vi "Get Plot visiblity.vi"(11 "Graph_refs":T2) -> (3 "Plot visibility":T1[](array[typedef]))   [LabVIEW 2018]
uses:
  Scope/controls/Graph_references.ctl
  Scope/controls/graph_controls.ctl
  Scope/controls/Plot visibility.ctl
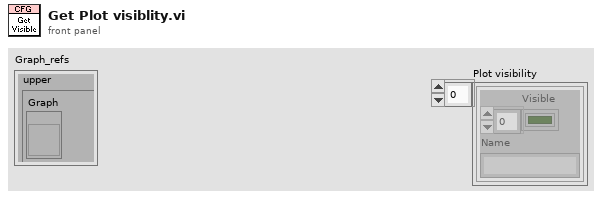
[diagram p1: front panel]
types:
  T1 = typedef "Plot visibility.ctl" = cluster{"Visible":bool[], "Name":string}
  T2 = typedef "Graph_references.ctl" = cluster{"upper":T3, "lower":T3, "Freq graph":refnum<vi>, "Adaptive FF graph":refnum<vi>}
  T3 = typedef "graph_controls.ctl" = cluster{"Graph":refnum<vi>, "Time btn":refnum<vi>, "Amplitude btn":refnum<vi>, "Chart":refnum<vi>}
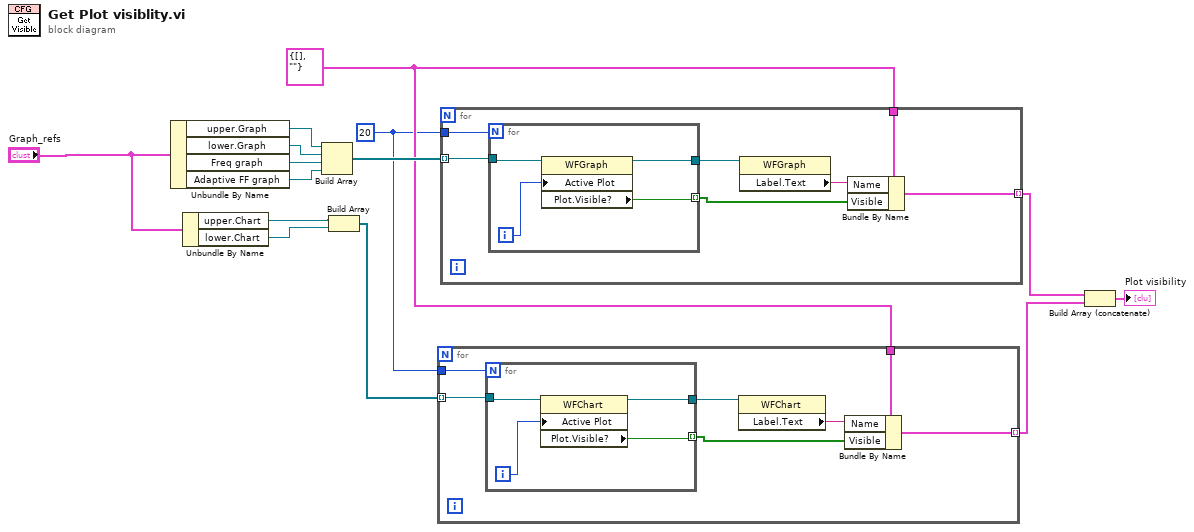
[diagram p0: block diagram]
diagram:
  w1 = 20
  w5 = T1 {"Visible"=[], "Name"=""} ("Plot visiblility")
  n1 = Unbundle By Name("Graph_refs") -> ("upper.Graph"=w14:refnum<vi>, "lower.Graph"=w13:refnum<vi>, "Freq graph"=w11:refnum<vi>, "Adaptive FF graph"=w10:refnum<vi>)
  n2 = Unbundle By Name("Graph_refs") -> ("upper.Chart"=w8:refnum<vi>, "lower.Chart"=w7:refnum<vi>)
  n3 = Build Array(w14, w13, w11, w10) -> (w12:refnum<vi>[])
  n4 = Build Array(w8, w7) -> (w6:refnum<vi>[])
  n5 = for {
    tunnel: w6 -> [w21] mode=indexing
    tunnel: w5 -> [w19]
    tunnel: [w16] -> w3 mode=indexing
    tunnel: w1 -> [w15]
    n6 = for {
      N: w15 -> [_]
      tunnel: w21 -> [w25]
      tunnel: [w23] -> w17 mode=indexing
      tunnel: [w22] -> w20
      i -> [w24]
      n7 = property on="Property Node" class="WFChart"(reference=w25, "Active Plot"=w24) -> (reference out=w22:refnum<vi>, "Plot.Visible?"=w23:bool)  [unwired: 1 in, 1 out]
    }
    n8 = property on="Property Node" class="WFChart"(reference=w20) -> ("Label.Text"=w18:string)  [unwired: 1 in, 2 out]
    n9 = Bundle By Name(cluster=w19, "Name"=w18, "Visible"=w17) -> (w16:T1)
  }
  n10 = for {
    tunnel: w12 -> [w32] mode=indexing
    tunnel: w5 -> [w30]
    tunnel: [w27] -> w4 mode=indexing
    tunnel: w1 -> [w26]
    n11 = for {
      N: w26 -> [_]
      tunnel: w32 -> [w36]
      tunnel: [w34] -> w28 mode=indexing
      tunnel: [w33] -> w31
      i -> [w35]
      n12 = property on="Property Node" class="WFGraph"(reference=w36, "Active Plot"=w35) -> (reference out=w33:refnum<vi>, "Plot.Visible?"=w34:bool)  [unwired: 1 in, 1 out]
    }
    n13 = property on="Property Node" class="WFGraph"(reference=w31) -> ("Label.Text"=w29:string)  [unwired: 1 in, 2 out]
    n14 = Bundle By Name(cluster=w30, "Name"=w29, "Visible"=w28) -> (w27:T1)
  }
  n15 = Build Array (concatenate)(w4, w3) -> (→"Plot visibility":T1[])
